vi "Digital Clock 2012 NIVerified.vi"() -> ()   [LabVIEW 2012]
uses:
  Black Display.ctl
  Vertical.ctl
  Horizontal.ctl
panel:
  out "Error Out":errorcluster caption="エラー出力"
  in  "Error In":errorcluster caption="エラー入力"
  out "Seconds":T1[](array[typedef])
  out "Minutes":T1[](array[typedef])
  out "Hours":T1[](array[typedef])
  in  "Stop Button":bool
  # "Overview: This application displays the real world current time as a digital display as you would see on an old digital alarm clock.\nRequirements: LabVIEW Base Development System 2012 (or compatible)\nInstructions: \n1. Run this VI."
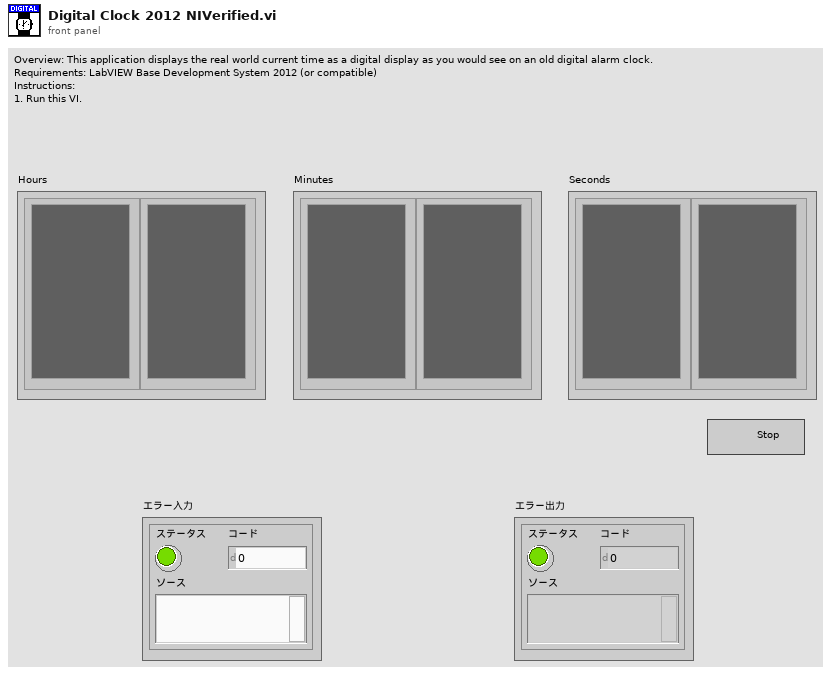
[diagram p1: front panel]
types:
  T1 = typedef "Black Display.ctl" = cluster{"V1":T2, "V2":T2, "H1":T3, "H2":T3, "V3":T2, "V4":T2, "H3":T3}
  T2 = typedef "Vertical.ctl" = bool
  T3 = typedef "Horizontal.ctl" = bool
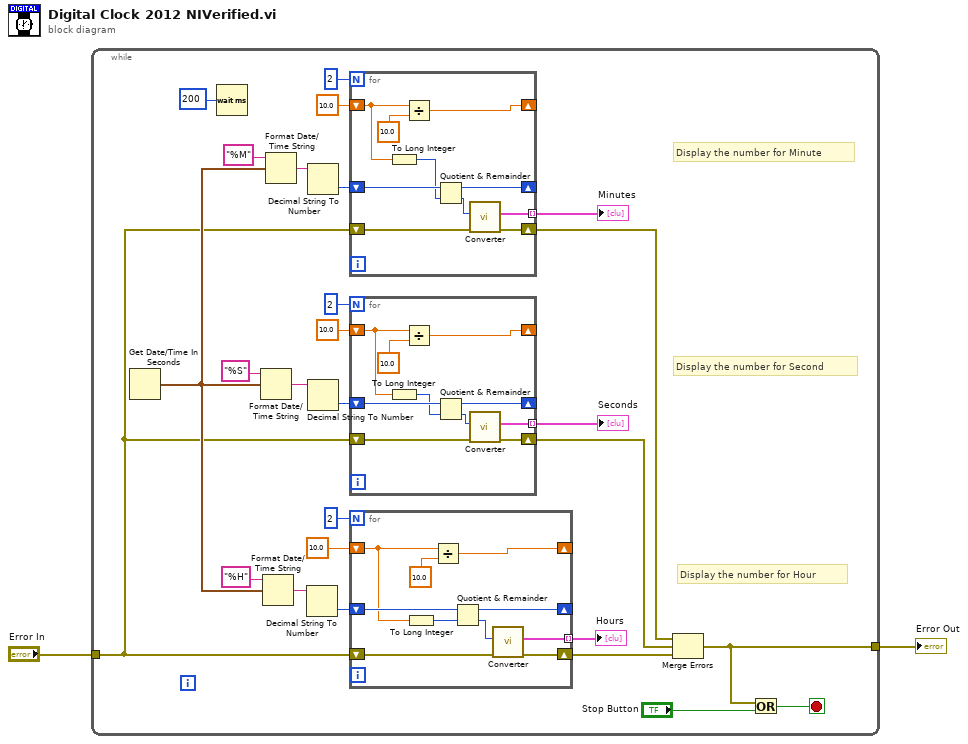
[diagram p0: block diagram]
diagram:
  n1 = while {
    tunnel: "Error In" -> [w7]
    tunnel: [w3] -> w1
    stop <- w9 stop-if-true
    # "Display the number for Hour"
    # "Display the number for Second"
    # "Display the number for Minute"
    n2 = Get Date/Time In Seconds() -> (seconds since 1Jan1904=w23:timestamp)
    n3 = Wait (ms)(milliseconds to wait=u32 200 ("millisecond multiple")) -> ()  [unwired: 1 out]
    n4 = Format Date/Time String(time format string (%c)="%S", seconds (now)=w23) -> (date/time string=w20:string)  [unwired: 1 in]
    n5 = Format Date/Time String(time format string (%c)="%H", seconds (now)=w23) -> (date/time string=w21:string)  [unwired: 1 in]
    n6 = Format Date/Time String(time format string (%c)="%M", seconds (now)=w23) -> (date/time string=w22:string)  [unwired: 1 in]
    n7 = Decimal String To Number(string=w21) -> (number=w19:i32)  [unwired: 2 in, 1 out]
    n8 = Decimal String To Number(string=w22) -> (number=w10:i32)  [unwired: 2 in, 1 out]
    n9 = Decimal String To Number(string=w20) -> (number=w11:i32)  [unwired: 2 in, 1 out]
    n10 = for {
      N: 2 ("Width") -> [_]
      tunnel: [w30] -> w28 mode=indexing
      shift-right: [w38] -> _
      shift-left: 10.0 ("x^y") -> [w36]
      shift-right: [w34] -> _
      shift-left: w10 -> [w37]
      shift-right: [w31] -> w5
      shift-left: w7 -> [w32]
      n11 = To Long Integer(number=w36) -> (32bit integer=w35:i32)
      n12 = Divide(x=w36, y=10.0) -> (x/y=w38:dbl)
      n13 = Quotient & Remainder(x=w37, y=w35) -> (x-y*floor(x/y)=w34:i32, floor(x/y)=w33:i32)
      n14 = call "Converter.vi"("Error In"=w32, "Numeric Control"=w33) -> ("Error Out"=w31:errorcluster, "Digit"=w30:T1)  [unwired: 8 in]
    }
    "Minutes" <- w28
    n15 = for {
      N: 2 ("Width") -> [_]
      tunnel: [w41] -> w27 mode=indexing
      shift-right: [w48] -> _
      shift-left: 10.0 ("x^y") -> [w46]
      shift-right: [w44] -> _
      shift-left: w11 -> [w47]
      shift-right: [w40] -> w4
      shift-left: w7 -> [w42]
      n16 = To Long Integer(number=w46) -> (32bit integer=w45:i32)
      n17 = Divide(x=w46, y=10.0) -> (x/y=w48:dbl)
      n18 = Quotient & Remainder(x=w47, y=w45) -> (x-y*floor(x/y)=w44:i32, floor(x/y)=w43:i32)
      n19 = call "Converter.vi"("Error In"=w42, "Numeric Control"=w43) -> ("Error Out"=w40:errorcluster, "Digit"=w41:T1)  [unwired: 8 in]
    }
    "Seconds" <- w27
    n20 = for {
      N: 2 ("Width") -> [_]
      tunnel: [w51] -> w29 mode=indexing
      shift-right: [w58] -> _
      shift-left: 10.0 ("x^y") -> [w56]
      shift-right: [w54] -> _
      shift-left: w19 -> [w57]
      shift-right: [w50] -> w6
      shift-left: w7 -> [w52]
      n21 = To Long Integer(number=w56) -> (32bit integer=w55:i32)
      n22 = Divide(x=w56, y=10.0) -> (x/y=w58:dbl)
      n23 = Quotient & Remainder(x=w57, y=w55) -> (x-y*floor(x/y)=w54:i32, floor(x/y)=w53:i32)
      n24 = call "Converter.vi"("Error In"=w52, "Numeric Control"=w53) -> ("Error Out"=w50:errorcluster, "Digit"=w51:T1)  [unwired: 8 in]
    }
    "Hours" <- w29
    n25 = Merge Errors(w5, w4, w6) -> (w3:errorcluster)
    n26 = Or(x=w3, y="Stop Button") -> (x .or. y?=w9:bool)
  }
  "Error Out" <- w1
